vi "Get SMO Serial Number.vi"(8 "error in (no error)":errorcluster, 11 "Inst.AH2500 in":refnum<class "Inst.AH2500.lvclass">) -> (0 "error out":errorcluster, 2 "Serial Number":string, 3 "Inst.AH2500 out":refnum<class "Inst.AH2500.lvclass">)   [LabVIEW 2019, in "Inst.AH2500.lvclass"]
doc: "Override this VI to return the serial number of your Instrument"
uses:
  Inst.AH2500.lvclass
  AH2500/AH2500.lvlib
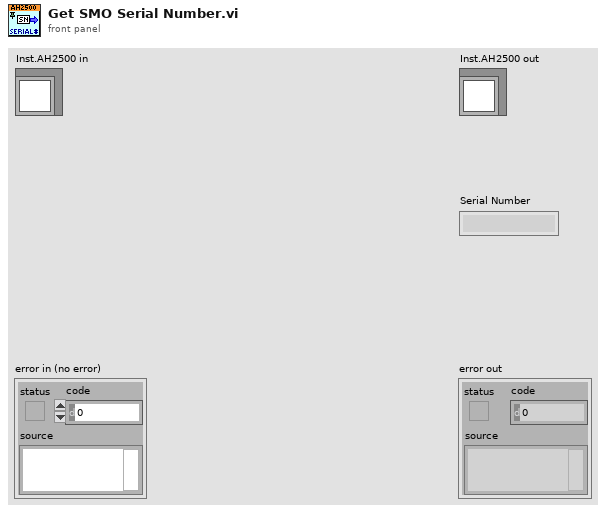
[diagram p1: front panel]
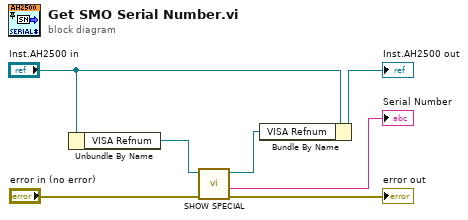
[diagram p0: block diagram]
diagram:
  n1 = Unbundle By Name("Inst.AH2500 in") -> ("VISA Refnum"=w7:refnum<visa-resource-name>)
  n2 = call "SHOW SPECIAL.vi"("error in (no error)"="error in (no error)", "VISA resource name"=w7) -> ("error out"=→"error out":errorcluster, "Serial Number"=→"Serial Number":string, "VISA resource name out"=w2:refnum<visa-resource-name>)  [unwired: 6 in, 1 out]
  n3 = Bundle By Name(cluster="Inst.AH2500 in", "VISA Refnum"=w2) -> (→"Inst.AH2500 out":refnum<class "Inst.AH2500.lvclass">)
